vi "Stopwatch, Reference.vi"(7 "Stop (Bool) Refnum":refnum<vi>, 8 "error in":errorcluster, 10 "Time Target (10s)":dbl[unit]=10.0 caption="Time Target (s)", 11 "Stopwatch (Knob) Refnum":refnum<vi>) -> (0 "error out":errorcluster {"code" format="%.0x"}, 2 "Time has Elapsed":bool, 3 "Elapsed Time":dbl[unit] format="%.2g")   [LabVIEW 2020]
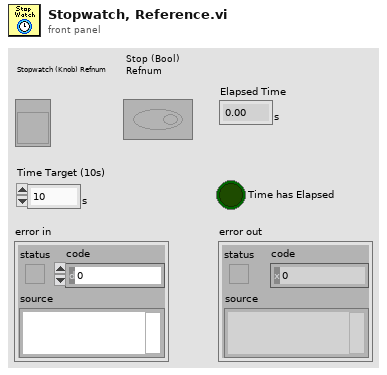
[diagram p1: front panel]
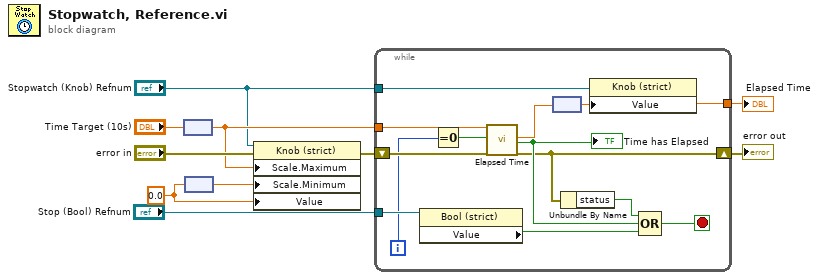
[diagram p0: block diagram]
diagram:
  w2 = dbl[unit] 0.0 ("Scale.Range:Minimum")
  n1 = node("Time Target (10s)") -> (w5:dbl)
  n2 = node(w2) -> (w3:dbl)
  n3 = property class="Knob (strict)"(reference="Stopwatch (Knob) Refnum", error in="error in", "Scale.Maximum"=w5, "Scale.Minimum"=w3, "Value"=w2) -> (error out=w6:errorcluster)  [unwired: 1 out]
  n4 = while {
    tunnel: w5 -> [w15]
    shift-right: [w19] -> w10
    shift-left: w6 -> [w22]
    tunnel: "Stopwatch (Knob) Refnum" -> [w18]
    tunnel: "Stop (Bool) Refnum" -> [w16]
    tunnel: [w13] -> w1
    i -> [w11]
    stop <- w21 stop-if-true
    n5 = property class="Bool (strict)"(reference=w16) -> ("Value"=w17:bool)  [unwired: 1 in, 2 out]
    n6 = Equal To 0?(x=w11) -> (x = 0?=w12:bool)
    n7 = call "Elapsed Time"("Time Target (s)"=w15, "Reset"=w12, "error in (no error)"=w22) -> ("Elapsed Time (s)"=w14:dbl, "Time has Elapsed"=w23:bool, "error out"=w19:errorcluster)  [unwired: 9 in, 5 out]
    "Time has Elapsed" <- w23
    n8 = node(w14) -> (w13:dbl[unit])
    n9 = Unbundle By Name(w19) -> ("status"=w20:bool)
    n10 = property class="Knob (strict)"(reference=w18, "Value"=w13) -> ()  [unwired: 1 in, 2 out]
    n11 = Compound Arithmetic op=OR(w20, w23, w17) -> (w21:bool)
  }
  "error out" <- w10
  "Elapsed Time" <- w1
